vi "Decode.vi"(8 "error in (no error)":errorcluster, 10 "Binary string in":string, 11 "obj in":refnum<class "AllInOne.lvclass">) -> (0 "error out":errorcluster, 1 "Data out":refnum<class "Data.lvclass">, 2 "Rest of binary string":string, 3 "obj out":refnum<class "AllInOne.lvclass">)   [LabVIEW 2020, in "AllInOne.lvclass"]
uses:
  AllInOne.lvclass
  Data Class/Data.lvclass
  Data Class/Datatypes/Data_AllInOne_class/Attribute.vi
  AllInOne.lvclass/AllInOne.ctl
  Data Class/Datatypes/Data_AllInOne_class/Data_AllInOne.lvclass
  C:/Users/theod/Desktop/API - EyeT data streaming to IC/Smart Eye API/Source/Classes/Smart Eye Pro Drivers/Data Class/Data.lvclass
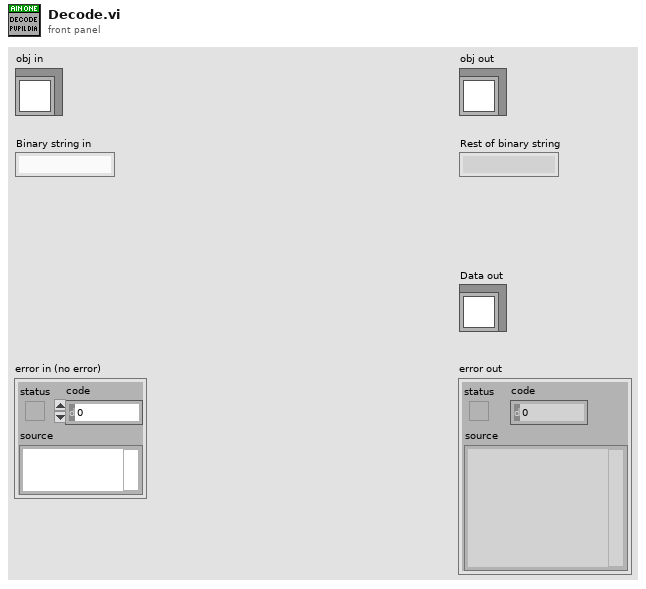
[diagram p1: front panel]
types:
  T1 = typedef "Data_AllInOne.lvclass/Attribute.vi" = cluster{"TimeStamp":u64, "FrameRate":dbl, "LeftPupilDiameter":dbl, "LeftPupilDiameterQ":dbl, "RightPupilDiameter":dbl, "RightPupilDiameterQ":dbl}
  T2 = enum16{"TimeStamp", "FrameRate", "LeftPupilDiameter", "LeftPupilDiameterQ", "RightPupilDiameter", "RightPupilDiameterQ"}[]
  T3 = enum16{"big-endian, network order", "native, host order", "little-endian"}
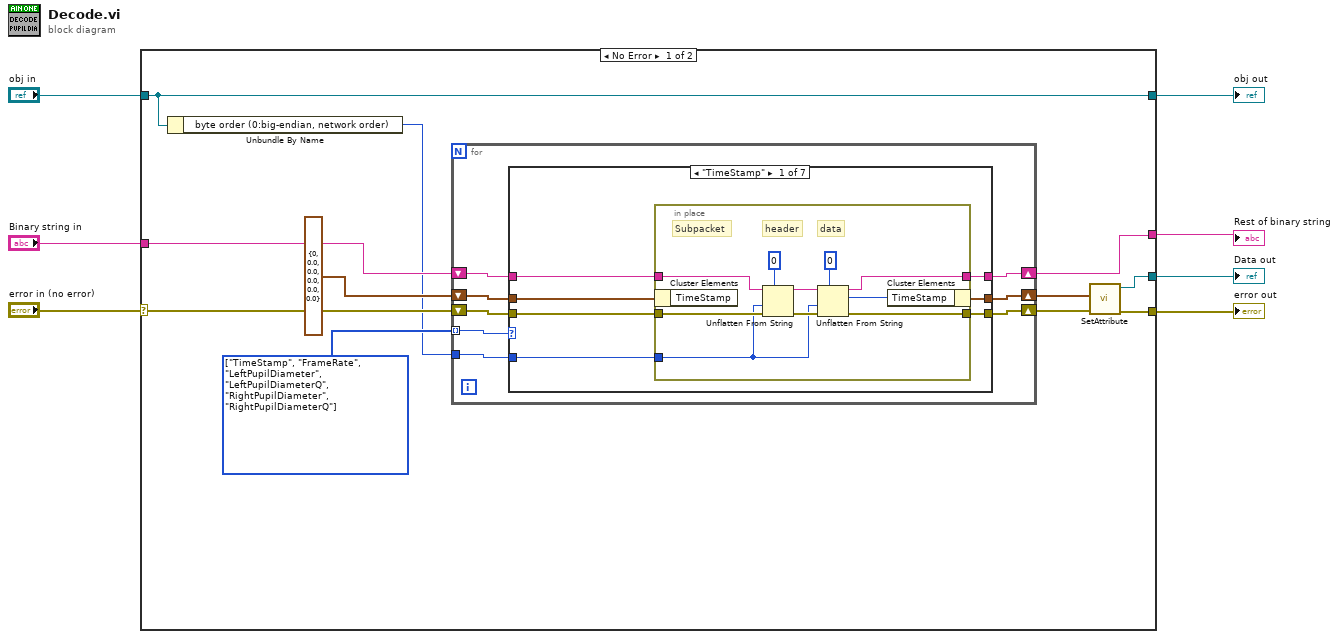
[diagram p0: block diagram]
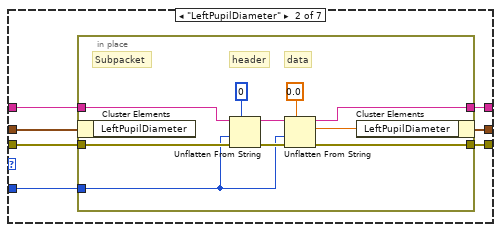
[diagram p2: hidden frame]
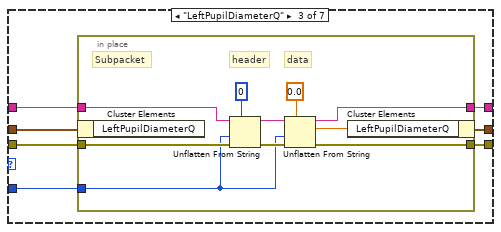
[diagram p3: hidden frame]
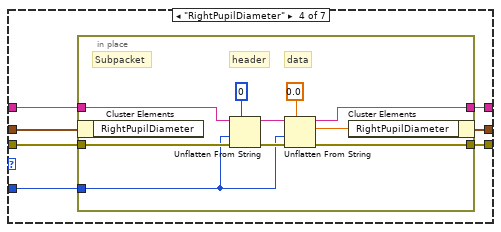
[diagram p4: hidden frame]
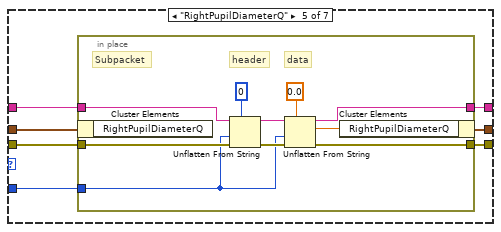
[diagram p5: hidden frame]
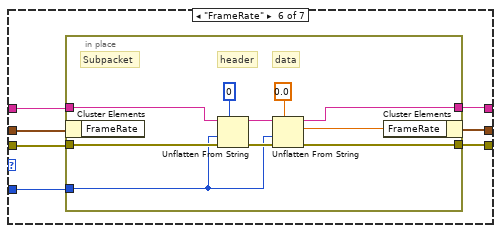
[diagram p6: hidden frame]
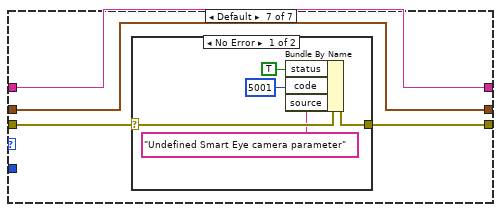
[diagram p7: hidden frame]
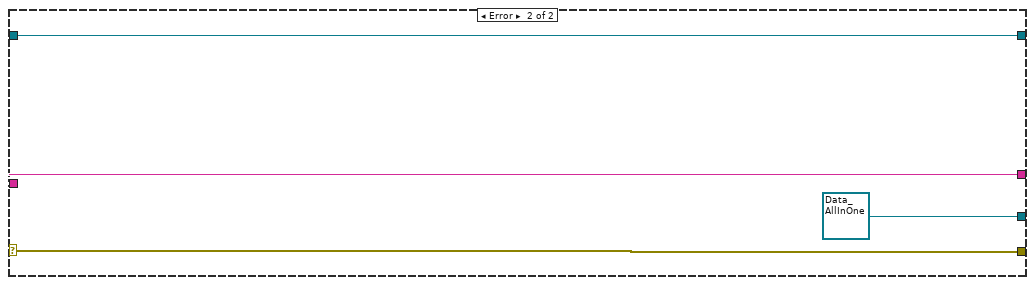
[diagram p9: hidden frame]
diagram:
  n1 = case shown="No Error" "error in (no error)" {
    selector: "error in (no error)" -> [w10 w142]
    tunnel: [w11 w142] -> w6
    tunnel: "obj in" -> [w9 w141]
    tunnel: [w9 w141] -> w4
    tunnel: "Binary string in" -> [w18 w140]
    tunnel: [w12 refnum<class "Data_AllInOne.lvclass"> refnum ("Data_Pupil_Diameter")] -> w2
    tunnel: [w15 w140] -> w1
    frame No Error {
      w16 = T2 [enum."TimeStamp", enum."FrameRate", enum."LeftPupilDiameter", enum."LeftPupilDiameterQ", enum."RightPupilDiameter", enum."RightPupilDiameterQ"] items=["TimeStamp", "FrameRate", "LeftPupilDiameter", "LeftPupilDiameterQ", "RightPupilDiameter", "RightPupilDiameterQ"]
      n2 = Unbundle By Name(w9) -> ("byte order (0:big-endian, network order)"=w8:T3)
      n3 = for {
        shift-right: [w23] -> w15
        shift-left: w18 -> [w24]
        shift-right: [w25] -> w14
        shift-left: T1 {"TimeStamp"=0, "FrameRate"=0.0, "LeftPupilDiameter"=0.0, "LeftPupilDiameterQ"=0.0, "RightPupilDiameter"=0.0, "RightPupilDiameterQ"=0.0} ("Attribute") -> [w26]
        tunnel: w16 -> [w22] mode=indexing
        shift-right: [w21] -> w13
        shift-left: w10 -> [w20]
        tunnel: w8 -> [w19]
        n4 = case shown="\"TimeStamp\"" w22 {
          tunnel: w26 -> [w33 w50 w67 w84 w101 w113 w130]
          tunnel: [w30 w47 w64 w81 w98 w117 w130] -> w25
          tunnel: w24 -> [w32 w49 w66 w83 w100 w112 w129]
          tunnel: [w31 w48 w65 w82 w99 w118 w129] -> w23
          tunnel: [w29 w46 w63 w80 w97 w116 w132] -> w21
          tunnel: w20 -> [w28 w45 w62 w79 w96 w114 w131]
          tunnel: w19 -> [w27 w44 w61 w78 w95 w115 _]
          frame "TimeStamp" {
            n5 = in-place {
              in-place-border: w32 -> [w40]
              in-place-border: [w39] -> w31
              in-place-border: [w38] -> w29
              in-place-border: w28 -> [w36]
              in-place-border: w27 -> [w35]
              # "header"
              # "data"
              # "Subpacket"
              n6 = in-place-cluster #1(w33) -> ()  [unwired: 1 out]
              n7 = Unflatten From String(type=0, binary string=w40, byte order (0:big-endian, network order)=w35, error in (no error)=w36) -> (rest of the binary string=w43:string, error out=w41:errorcluster)  [unwired: 1 in, 1 out]
              n8 = Unflatten From String(type=u64 0, binary string=w43, byte order (0:big-endian, network order)=w35, error in (no error)=w41) -> (rest of the binary string=w39:string, value=w34:u64, error out=w38:errorcluster)  [unwired: 1 in]
              n9 = in-place-cluster #1("TimeStamp"=w34) -> (w30:T1)
            }
          }
          frame "LeftPupilDiameter" {
            n10 = in-place {
              in-place-border: w49 -> [w57]
              in-place-border: [w56] -> w48
              in-place-border: [w55] -> w46
              in-place-border: w45 -> [w53]
              in-place-border: w44 -> [w51]
              # "header"
              # "data"
              # "Subpacket"
              n11 = in-place-cluster #2(w50) -> ()  [unwired: 1 out]
              n12 = Unflatten From String(type=0, binary string=w57, byte order (0:big-endian, network order)=w51, error in (no error)=w53) -> (rest of the binary string=w60:string, error out=w58:errorcluster)  [unwired: 1 in, 1 out]
              n13 = Unflatten From String(type=0.0, binary string=w60, byte order (0:big-endian, network order)=w51, error in (no error)=w58) -> (rest of the binary string=w56:string, value=w52:dbl, error out=w55:errorcluster)  [unwired: 1 in]
              n14 = in-place-cluster #2("LeftPupilDiameter"=w52) -> (w47:T1)
            }
          }
          frame "LeftPupilDiameterQ" {
            n15 = in-place {
              in-place-border: w66 -> [w74]
              in-place-border: [w73] -> w65
              in-place-border: [w72] -> w63
              in-place-border: w62 -> [w70]
              in-place-border: w61 -> [w68]
              # "header"
              # "data"
              # "Subpacket"
              n16 = in-place-cluster #3(w67) -> ()  [unwired: 1 out]
              n17 = Unflatten From String(type=0, binary string=w74, byte order (0:big-endian, network order)=w68, error in (no error)=w70) -> (rest of the binary string=w77:string, error out=w75:errorcluster)  [unwired: 1 in, 1 out]
              n18 = Unflatten From String(type=0.0, binary string=w77, byte order (0:big-endian, network order)=w68, error in (no error)=w75) -> (rest of the binary string=w73:string, value=w69:dbl, error out=w72:errorcluster)  [unwired: 1 in]
              n19 = in-place-cluster #3("LeftPupilDiameterQ"=w69) -> (w64:T1)
            }
          }
          frame "RightPupilDiameter" {
            n20 = in-place {
              in-place-border: w83 -> [w91]
              in-place-border: [w90] -> w82
              in-place-border: [w89] -> w80
              in-place-border: w79 -> [w87]
              in-place-border: w78 -> [w85]
              # "header"
              # "data"
              # "Subpacket"
              n21 = in-place-cluster #4(w84) -> ()  [unwired: 1 out]
              n22 = Unflatten From String(type=0, binary string=w91, byte order (0:big-endian, network order)=w85, error in (no error)=w87) -> (rest of the binary string=w94:string, error out=w92:errorcluster)  [unwired: 1 in, 1 out]
              n23 = Unflatten From String(type=0.0, binary string=w94, byte order (0:big-endian, network order)=w85, error in (no error)=w92) -> (rest of the binary string=w90:string, value=w86:dbl, error out=w89:errorcluster)  [unwired: 1 in]
              n24 = in-place-cluster #4("RightPupilDiameter"=w86) -> (w81:T1)
            }
          }
          frame "RightPupilDiameterQ" {
            n25 = in-place {
              in-place-border: w100 -> [w108]
              in-place-border: [w107] -> w99
              in-place-border: [w106] -> w97
              in-place-border: w96 -> [w104]
              in-place-border: w95 -> [w102]
              # "header"
              # "data"
              # "Subpacket"
              n26 = in-place-cluster #5(w101) -> ()  [unwired: 1 out]
              n27 = Unflatten From String(type=0, binary string=w108, byte order (0:big-endian, network order)=w102, error in (no error)=w104) -> (rest of the binary string=w111:string, error out=w109:errorcluster)  [unwired: 1 in, 1 out]
              n28 = Unflatten From String(type=0.0, binary string=w111, byte order (0:big-endian, network order)=w102, error in (no error)=w109) -> (rest of the binary string=w107:string, value=w103:dbl, error out=w106:errorcluster)  [unwired: 1 in]
              n29 = in-place-cluster #5("RightPupilDiameterQ"=w103) -> (w98:T1)
            }
          }
          frame "FrameRate" {
            n30 = in-place {
              in-place-border: w112 -> [w125]
              in-place-border: [w124] -> w118
              in-place-border: [w123] -> w116
              in-place-border: w114 -> [w121]
              in-place-border: w115 -> [w119]
              # "header"
              # "data"
              # "Subpacket"
              n31 = in-place-cluster #6(w113) -> ()  [unwired: 1 out]
              n32 = Unflatten From String(type=0, binary string=w125, byte order (0:big-endian, network order)=w119, error in (no error)=w121) -> (rest of the binary string=w128:string, error out=w126:errorcluster)  [unwired: 1 in, 1 out]
              n33 = Unflatten From String(type=0.0, binary string=w128, byte order (0:big-endian, network order)=w119, error in (no error)=w126) -> (rest of the binary string=w124:string, value=w120:dbl, error out=w123:errorcluster)  [unwired: 1 in]
              n34 = in-place-cluster #6("FrameRate"=w120) -> (w117:T1)
            }
          }
          frame Default {
            n35 = case shown="No Error" w131 {
              selector: w131 -> [w136 w138]
              tunnel: [w137 w138] -> w132
              frame No Error {
                n36 = Bundle By Name(cluster=w136, "status"=TRUE, "code"=5001, "source"="Undefined Smart Eye camera parameter") -> (w137:errorcluster)
              }
              frame Error {
              }
            }
          }
        }
      }
      n37 = call "SetAttribute.vi"("error in (no error)"=w13, "Set Attribute"=w14) -> ("error out"=w11:errorcluster, "Data_AllInOne out"=w12:refnum<class "Data_AllInOne.lvclass">)  [unwired: 8 in]
    }
    frame Error {
    }
  }
  "error out" <- w6
  "obj out" <- w4
  "Data out" <- w2
  "Rest of binary string" <- w1
